vi "PMT_plus_Kiethley2450_and_2410.vi"() -> ()   [LabVIEW 2022 SP3]
uses:
  <vilib>/Utility/file.llb/Write Delimited Spreadsheet (string).vi
  <vilib>/Analysis/1siggen.llb/Ramp Pattern by Delta.vi
  <vilib>/Utility/file.llb/Write Delimited Spreadsheet (DBL).vi
  <vilib>/Analysis/NI_AALBase.lvlib
  C:/Users/Public/OneDrive/Desktop/test_save_lv22/Close.vi/Close Folder/Users/Public/OneDrive/Desktop/Keithley_2450_2470_1_4_0_LV2015_NewReadme2_2450-LV2015-1.4.0/Keithley 2450/Keithley 2450.lvlib
  D:/Download/Keithley 24XX/Keithley 24XX Folder/D/Download/Keithley 24XX/Keithley 24XX.lvlib
panel:
  out "current E field":dbl
  in  "d_t":dbl=-1.0 format="%#_13g"
  in  "d_b":dbl=-1.0 format="%#_13g"
  in  "E step (V/nm)":dbl=0.5 format="%#_13g"
  in  "E end (V/nm)":dbl=-1.0 format="%#_13g"
  in  "E start (V/nm)":dbl format="%#_13g"
  in  "Loop?":bool
  out "error out":errorcluster
  in  "use 2410":bool
  in  "use 2450?":bool=TRUE
  out "Set voltage 2410":dbl=-0.0
  out "current 2450":dbl=2.5622937e-12 format="%e"
  out "actual voltage 2410":dbl format="%0.2f"
  out "current 2410":dbl format="%e"
  in  "Compliance  Level 2410 (0.1)":dbl=1e-08
  in  "VISA resource name 2410":refnum<visa-resource-name>
  out "Serial Configuration":T1={"Baud Rate"=9600, "Parity"=0, "Data Bits"=8, "Stop Bits"=10, "Flow Control"=0} {"Flow Control" items=["None", "XON/XOFF", "RTS/CTS", "XON/XOFF & RTS/CTS", "DTR/DSR", "XON/XOFF & DTR/DSR"]; "Stop Bits" items=["1.0"=10, "1.5"=15, "2.0"=20]; "Data Bits" items=["7"=7, "8"=8]; "Parity" items=["None", "Odd", "Even", "Mark", "Space"]; "Baud Rate" items=["300"=300, "600"=600, "1200"=1200, "2400"=2400, "4800"=4800, "9600"=9600, "19200"=19200]}
  in  "Use PMT?":bool=TRUE
  out "XY Graph":cluster{dbl[], dbl[]}(graph)={[-1.0, -0.5, 0.0], [45.5, 47.5, 49.0]}
  out "Actual Voltage 2450":dbl
  in  "Num Current Meas":i32=20
  in  "Path":path=path "C:/Users/Public/OneDrive/Desktop/test.txt"
  in  "error in (no error)":errorcluster
  in  "VISA resource name":refnum<visa-resource-name>="GPIB0::1::INSTR"
  out "Set Voltage 2450":dbl
  in  "Step Size (V)":dbl=0.5 format="%#_13g"
  in  "End V":dbl=-1.0 format="%#_13g"
  in  "Start V":dbl format="%#_13g"
  in  "Source Limit Level (0.1)":dbl=1e-08
  out "standard deviation":dbl
  out "mean":dbl=49.0
  out "data":u32[](array[numeric])=[49, 49]
  out "OLD":bool
  out "DB":u32[](array[numeric])=[49, 0, 0, 0, 0, 0, 0, 0, 0, 0, 0, 0, 0, 0, 0, 0]
  out "Overload":i32
  out "Gate Number":i32=1
  in  "Correction":bool=TRUE
  out "Num Gates Read":i32=2
  out "Gate Time Read":i32=100 caption="Gate time Read"
  out "Num Gates Set":i32=2
  out "Gate Time Set":i32=100
  out "PowerD":i32 caption="Power\nRead Data"
  out "Handle Number":i32=173123648
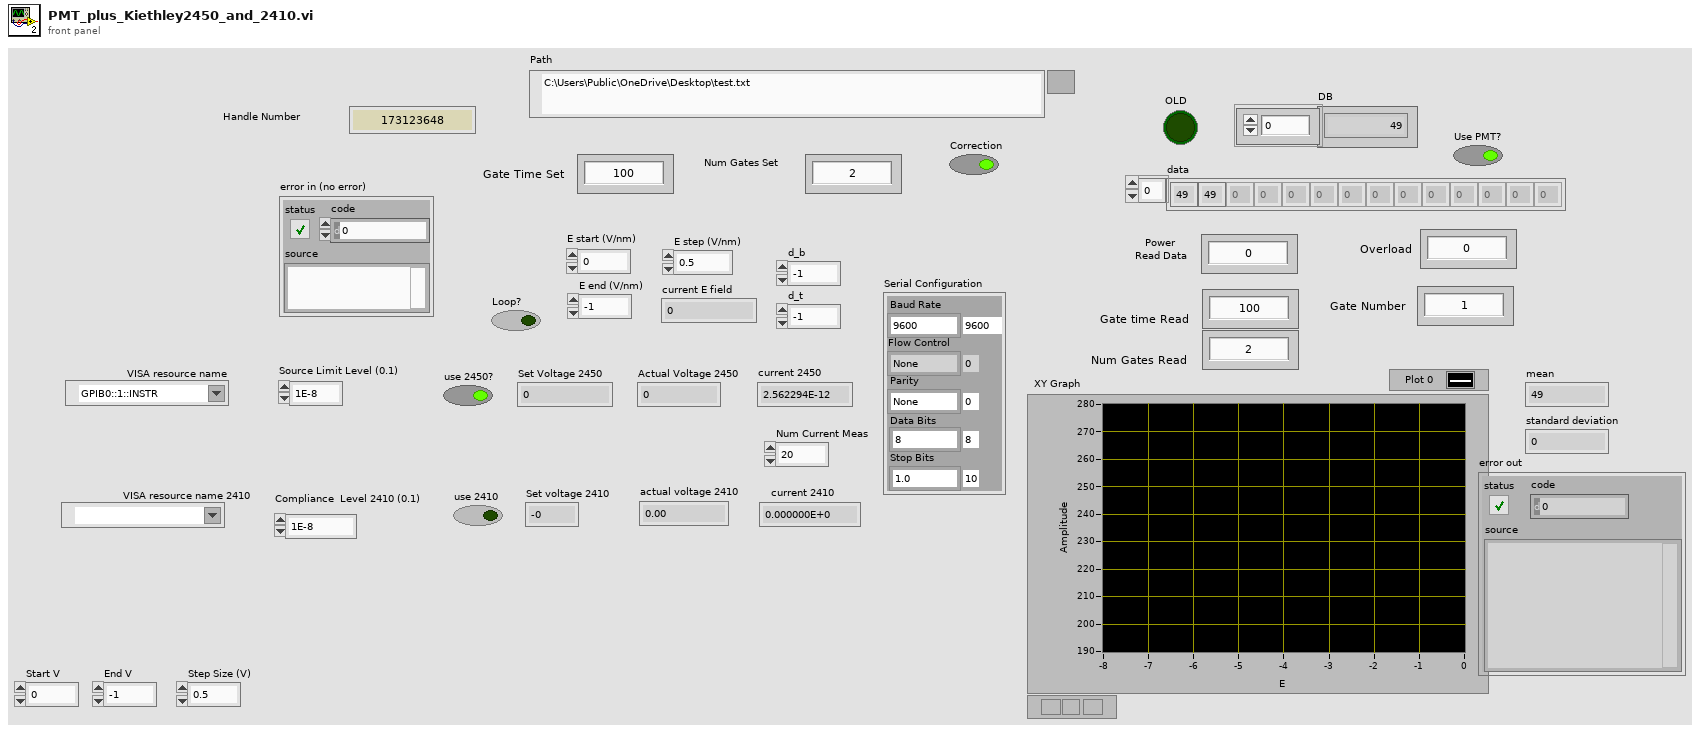
[diagram p1: front panel]
types:
  T1 = cluster{"Baud Rate":u32, "Parity":u16, "Data Bits":u16, "Stop Bits":u16, "Flow Control":u16}
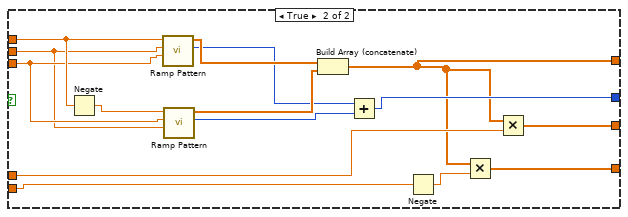
[diagram p2: hidden frame]
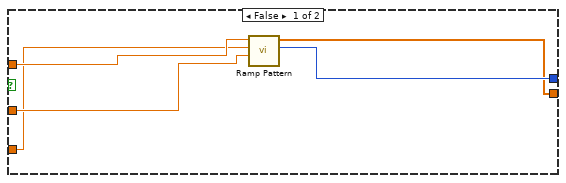
[diagram p3: hidden frame]
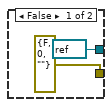
[diagram p4: hidden frame]
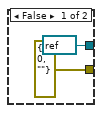
[diagram p5: hidden frame]
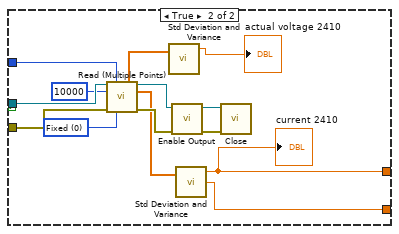
[diagram p6: hidden frame]
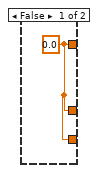
[diagram p7: hidden frame]
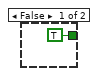
[diagram p8: hidden frame]
diagram:
  n1 = flat-sequence {
    tunnel: [w27] -> w8
    tunnel: [w15] -> w7
    tunnel: ["Path"] -> w5
    tunnel: ["use 2410"] -> w4
    tunnel: [w11] -> w3
    tunnel: [w10] -> w2
    tunnel: [w9] -> w1
    tunnel: w8 -> [w93]
    tunnel: w7 -> [w92]
    tunnel: [w91] -> w6
    tunnel: w5 -> [w90]
    tunnel: w4 -> [w85]
    tunnel: w3 -> [w84]
    tunnel: w2 -> [w83]
    tunnel: w1 -> [w82]
    tunnel: w6 -> [w575]
    frame #0 {
      # "open PMT and turn on power"
      n2 = call "Open.vi"("Serial Number"="30430219") -> ("Handle Number"=w31:i32)  [unwired: 9 in, 1 out]
      "Handle Number" <- w31
      n3 = case shown="False" "Loop?" {
        tunnel: "E step (V/nm)" -> [w46 w61]
        tunnel: "E end (V/nm)" -> [w45 w58]
        tunnel: "E start (V/nm)" -> [w44 w59]
        tunnel: [w43 w55] -> w15
        tunnel: "d_t" -> [w38 w49]
        tunnel: "d_b" -> [w42 w52]
        tunnel: [w41 w51] -> w11
        tunnel: [w40 w50] -> w10
        tunnel: [w37 w47] -> w9
        frame False {
          n4 = call-poly <vilib>:"Ramp Pattern.vi"("start"=w44, "end"=w45, "delta"=w46) -> ("samples"=w43:i32, "Ramp Pattern"=w37:dbl[])  [unwired: 6 in, 1 out]
          n5 = Negate(x=w38) -> (-x=w39:dbl)
          n6 = Multiply(x=w37, y=w39) -> (x*y=w40:dbl[])
          n7 = Multiply(x=w37, y=w42) -> (x*y=w41:dbl[])
        }
        frame True {
          n8 = Negate(x=w61) -> (-x=w60:dbl)
          n9 = call-poly <vilib>:"Ramp Pattern.vi"("start"=w59, "end"=w58, "delta"=w61) -> ("samples"=w54:i32, "Ramp Pattern"=w57:dbl[])  [unwired: 6 in, 1 out]
          n10 = call-poly <vilib>:"Ramp Pattern.vi"("start"=w58, "end"=w59, "delta"=w60) -> ("samples"=w53:i32, "Ramp Pattern"=w56:dbl[])  [unwired: 6 in, 1 out]
          n11 = Build Array (concatenate)(w57, w56) -> (w47:dbl[])
          n12 = Add(x=w54, y=w53) -> (x+y=w55:i32)
          n13 = Negate(x=w49) -> (-x=w48:dbl)
          n14 = Multiply(x=w47, y=w48) -> (x*y=w50:dbl[])
          n15 = Multiply(x=w47, y=w52) -> (x*y=w51:dbl[])
        }
      }
      n16 = Boolean To (0,1)(Boolean="Use PMT?") -> (0, 1=w32:i16)
      n17 = call "Read HV.vi"("handle"=w31) -> ("HV out"=w30:i32, "handle out"=w34:i32)  [unwired: 8 in, 1 out]
      n18 = case shown="True" "Loop?" {
        tunnel: "Start V" -> [w63 w74]
        tunnel: "End V" -> [w62 w72]
        tunnel: [w65 w71] -> _
        tunnel: [w66 w70] -> _
        tunnel: "Step Size (V)" -> [w64 w68]
        frame False {
          n19 = call-poly <vilib>:"Ramp Pattern.vi"("start"=w63, "end"=w62, "delta"=w64) -> ("samples"=w66:i32, "Ramp Pattern"=w65:dbl[])  [unwired: 6 in, 1 out]
        }
        frame True {
          w69 = -1.0
          n20 = Multiply(x=w68, y=w69) -> (x*y=w67:dbl)
          n21 = Multiply(x=w72, y=w69) -> (x*y=w73:dbl)
          n22 = call-poly <vilib>:"Ramp Pattern.vi"("start"=w74, "end"=w72, "delta"=w68) -> ("samples"=w78:i32, "Ramp Pattern"=w75:dbl[])  [unwired: 6 in, 1 out]
          n23 = call-poly <vilib>:"Ramp Pattern.vi"("start"=w73, "end"=w74, "delta"=w68) -> ("samples"=w81:i32, "Ramp Pattern"=w77:dbl[])  [unwired: 6 in, 1 out]
          n24 = call-poly <vilib>:"Ramp Pattern.vi"("start"=w72, "end"=w73, "delta"=w67) -> ("samples"=w79:i32, "Ramp Pattern"=w76:dbl[])  [unwired: 6 in, 1 out]
          n25 = Add(x=w78, y=w79) -> (x+y=w80:i32)
          n26 = Build Array (concatenate)(w75, w76, w77) -> (w71:dbl[])
          n27 = Add(x=w80, y=w81) -> (x+y=w70:i32)
        }
      }
      n28 = local write "PowerD"(w30) -> ()
      n29 = To Long Integer(number=w32) -> (32bit integer=w33:i32)
      n30 = call "Set HV.vi"("HV"=w33, "handle"=w34) -> ("handle out"=w36:i32)  [unwired: 8 in, 1 out]
      n31 = call "Read HV.vi"("handle"=w36) -> ("HV out"=w35:i32, "handle out"=w27:i32)  [unwired: 8 in, 1 out]
      n32 = Build Array("# SetVoltage2450(V) ActualVoltage2450(V) CountsMean CountsStd Current2450(uA) Current2450Std(uA) Current2410(uA) Current2410Std(uA)") -> (w22:string[])
      n33 = local write "PowerD"(w35) -> ()
      n34 = call-poly <vilib>:"Write Delimited Spreadsheet.vi"("file path (dialog if empty)"="Path", "1D data"=w22, "append to file? (new file:F)"=TRUE) -> ()  [unwired: 11 in, 2 out]
    }
    frame #1 {
      w88 = 0
      w89 = 0
      n35 = Initialize Array(w88, w88) -> (w87:i32[])
      n36 = Initialize Array(w89, w89) -> (w86:i32[])
      n37 = for {
        N: w92 -> [_]
        tunnel: w84 -> [w136] mode=indexing
        tunnel: w93 -> [w135]
        tunnel: [w134] -> w91
        tunnel: w90 -> [w133]
        shift-right: [w120] -> _
        shift-left: w86 -> [w128]
        shift-right: [w121] -> _
        shift-left: w87 -> [w127]
        tunnel: w85 -> [w98]
        tunnel: w83 -> [w95] mode=indexing
        tunnel: w82 -> [w94] mode=indexing
        n38 = flat-sequence {
          tunnel: w127 -> [w153]
          tunnel: w128 -> [w154]
          tunnel: w136 -> [w142]
          tunnel: [w142] -> w119
          tunnel: [w154] -> w117
          tunnel: [w153] -> w115
          tunnel: [w149] -> w113
          tunnel: [w148] -> w111
          tunnel: [w145] -> w107
          tunnel: [w144] -> w105
          tunnel: ["Num Current Meas"] -> w103
          tunnel: ["use 2450?"] -> w99
          tunnel: w98 -> [w138]
          tunnel: [w138] -> w96
          tunnel: w95 -> [w137]
          tunnel: w119 -> [w217]
          tunnel: [w217] -> w118
          tunnel: w117 -> [w216]
          tunnel: [w216] -> w116
          tunnel: w115 -> [w215]
          tunnel: [w215] -> w114
          tunnel: w113 -> [w214]
          tunnel: [w214] -> w112
          tunnel: w111 -> [w213]
          tunnel: [w213] -> w110
          tunnel: [w212] -> w108
          tunnel: w107 -> [w212]
          tunnel: [w211] -> w106
          tunnel: w105 -> [w211]
          tunnel: [w210] -> w104
          tunnel: w103 -> [w210]
          tunnel: [w209] -> w100
          tunnel: w99 -> [w209]
          tunnel: [w208] -> w97
          tunnel: w96 -> [w208]
          tunnel: [w231] -> w132
          tunnel: [w232] -> w131
          tunnel: [w222] -> w130
          tunnel: [w231] -> w129
          tunnel: [w230] -> w126
          tunnel: [w229] -> w125
          tunnel: w118 -> [w231]
          tunnel: w116 -> [w230]
          tunnel: w114 -> [w229]
          tunnel: w112 -> [w225]
          tunnel: w110 -> [w226]
          tunnel: [w223] -> w109
          tunnel: w108 -> [w228]
          tunnel: w106 -> [w227]
          tunnel: w104 -> [w224]
          tunnel: [w221] -> w102
          tunnel: [w220] -> w101
          tunnel: w100 -> [w219]
          tunnel: w97 -> [w218]
          tunnel: w135 -> [w289]
          tunnel: w133 -> [w287]
          tunnel: w132 -> [w286]
          tunnel: w131 -> [w285]
          tunnel: w130 -> [w284]
          tunnel: w129 -> [w282]
          tunnel: w126 -> [w281]
          tunnel: w125 -> [w280]
          tunnel: [w288] -> w124
          tunnel: [w279] -> w123
          tunnel: [w278] -> w122
          tunnel: w109 -> [w277]
          tunnel: w102 -> [w275]
          tunnel: w101 -> [w274]
          tunnel: [w572] -> w120
          tunnel: [w573] -> w121
          tunnel: [w574] -> w134
          tunnel: w124 -> [w574]
          tunnel: w123 -> [w573]
          tunnel: w122 -> [w572]
          frame #0 {
            w140 = TRUE
            w146 = FALSE
            n39 = case shown="True" "use 2450?" {
              tunnel: "VISA resource name" -> [_ w198]
              tunnel: "error in (no error)" -> [_ w197]
              tunnel: TRUE -> [_ w193]
              tunnel: [errorcluster {"status"=FALSE, "code"=0, "source"=""} ("error out") w192] -> w149
              tunnel: [refnum<visa-resource-name> refnum ("VISA resource name out") w191] -> w148
              tunnel: w146 -> [_ w190]
              tunnel: "Num Current Meas" -> [_ w181]
              tunnel: w142 -> [_ w180]
              tunnel: "Source Limit Level (0.1)" -> [_ w179]
              tunnel: w140 -> [_ w178]
              tunnel: w140 -> [_ w177]
              frame False {
              }
              frame True {
                w194 = 1
                w196 = 0
                n40 = call "Initialize.vi"("error in (no error)"=w197, "Reset (True)"=w190, "ID Query (True)"=w193, "VISA resource name"=w198) -> ("error out"=w188:errorcluster, "VISA resource name out"=w189:refnum<visa-resource-name>)  [unwired: 6 in]
                n41 = call "Clear Buffer.vi"("VISA resource name"=w189, "error in (no error)"=w188) -> ("VISA resource name out"=w186:refnum<visa-resource-name>, "error out"=w187:errorcluster)  [unwired: 12 in]
                n42 = call "Configure Measurement Range.vi"("error in (no error)"=w187, "Enable Auto Range (T:Enable)"=w177, "Function (0: Volts)"=w196, "VISA resource name"=w186) -> ("error out"=w206:errorcluster, "VISA resource name out"=w205:refnum<visa-resource-name>)  [unwired: 6 in]
                n43 = call "Configure Measurement Range.vi"("error in (no error)"=w206, "Enable Auto Range (T:Enable)"=w178, "Function (0: Volts)"=w194, "VISA resource name"=w205) -> ("error out"=w202:errorcluster, "VISA resource name out"=w199:refnum<visa-resource-name>)  [unwired: 6 in]
                n44 = call "Configure Output.vi"("VISA resource name"=w199, "Source Level (0)"=w180, "Source Limit Level (0.1)"=w179, "error in (no error)"=w202) -> ("VISA resource name out"=w200:refnum<visa-resource-name>, "error out"=w203:errorcluster)  [unwired: 10 in]
                n45 = call "Configure Source Function.vi"("error in (no error)"=w203, "Function (0: Volts)"=w196, "VISA resource name"=w200) -> ("error out"=w204:errorcluster, "VISA resource name out"=w201:refnum<visa-resource-name>)  [unwired: 7 in]
                n46 = call "Configure Measurement Function.vi"("error in (no error)"=w204, "Function (0: Volts)"=w194, "VISA resource name"=w201) -> ("error out"=w182:errorcluster, "VISA resource name out"=w185:refnum<visa-resource-name>)  [unwired: 7 in]
                n47 = call "Set Measurement Count.vi"("error in (no error)"=w182, "Measurement Count (1)"=w181, "VISA resource name"=w185) -> ("error out"=w183:errorcluster, "VISA resource name out"=w184:refnum<visa-resource-name>)  [unwired: 7 in]
                n48 = call "Enable Output.vi"("error in (no error)"=w183, "Enable Output (T: Enable)"=TRUE, "VISA resource name"=w184) -> ("error out"=w192:errorcluster, "VISA resource name out"=w191:refnum<visa-resource-name>)  [unwired: 7 in]
              }
            }
            n49 = case shown="True" w138 {
              tunnel: "VISA resource name 2410" -> [_ w174]
              tunnel: w146 -> [_ w173]
              tunnel: [refnum<visa-resource-name> refnum ("VISA resource name out") w160] -> w145
              tunnel: [errorcluster {"status"=FALSE, "code"=0, "source"=""} ("error out") w159] -> w144
              tunnel: w137 -> [_ w158]
              tunnel: w140 -> [_ w157]
              frame False {
              }
              frame True {
                w162 = u16 0 items=["Voltage", "Current"] ("Source Mode  (0: Voltage)")
                w163 = u16 1 items=["Volts", "Current", "Resistance"] ("Function (0: Volts)")
                w164 = u16 0 items=["Volts", "Current", "Resistance"] ("Function (0: Volts)")
                n50 = call "Initialize.vi"("Reset (True)"=w173, "VISA resource name"=w174) -> ("error out"=w171:errorcluster, "VISA resource name out"=w172:refnum<visa-resource-name>)  [unwired: 8 in]
                n51 = call "Configure Measurement.vi"("error in (no error)"=w171, "Enable Auto Range (T:Enable)"=w157, "Function (0: Volts)"=w164, "VISA resource name"=w172) -> ("error out"=w170:errorcluster, "VISA resource name out"=w169:refnum<visa-resource-name>)  [unwired: 6 in]
                n52 = call "Configure Measurement.vi"("error in (no error)"=w170, "Enable Auto Range (T:Enable)"=w157, "Function (0: Volts)"=w163, "VISA resource name"=w169) -> ("error out"=w167:errorcluster, "VISA resource name out"=w168:refnum<visa-resource-name>)  [unwired: 6 in]
                n53 = call "Configure Output.vi"("Source Mode  (0: Voltage)"=w162, "error in (no error)"=w167, "Compliance  Level (0.1)"="Compliance  Level 2410 (0.1)", "Output Level (0)"=w158, "VISA resource name"=w168) -> ("error out"=w165:errorcluster, "VISA resource name out"=w166:refnum<visa-resource-name>)  [unwired: 5 in]
                n54 = call "Enable Output.vi"("error in (no error)"=w165, "VISA resource name"=w166) -> ("error out"=w159:errorcluster, "VISA resource name out"=w160:refnum<visa-resource-name>)  [unwired: 8 in]
              }
            }
            "Set Voltage 2450" <- w142
            "Set voltage 2410" <- w137
          }
          frame #1 {
            n55 = Wait (ms)(milliseconds to wait=u32 100) -> ()  [unwired: 1 out]
          }
          frame #2 {
            n56 = case shown="False" w218 {
              tunnel: w228 -> [_ w247]
              tunnel: w227 -> [_ w246]
              tunnel: w224 -> [_ w237]
              tunnel: [w233 w235] -> w221
              tunnel: [w233 w234] -> w220
              frame False {
                w233 = 0.0 ("mean")
              }
              frame True {
                w245 = u16 0 items=["Fixed", "Sweep", "List"] ("Output Mode (0: Fixed)")
                n57 = call "Read (Multiple Points).vi"("VISA resource name"=w247, "Sample Count (1)"=w237, "Timeout (10000 ms)"=10000, "error in (no error)"=w246, "Output Mode (0: Fixed)"=w245) -> ("Voltage"=w238:sgl[], "VISA resource name out"=w243:refnum<visa-resource-name>, "Current"=w239:sgl[], "error out"=w240:errorcluster)  [unwired: 4 in, 3 out]
                n58 = call <vilib>:"Std Deviation and Variance.vi"("X"=w238) -> ("mean"=→"actual voltage 2410":dbl)  [unwired: 1 in, 2 out]
                n59 = call "Enable Output.vi"("error in (no error)"=w240, "VISA resource name"=w243) -> ("error out"=w241:errorcluster, "VISA resource name out"=w242:refnum<visa-resource-name>)  [unwired: 8 in]
                n60 = call <vilib>:"Std Deviation and Variance.vi"("X"=w239) -> ("mean"=w235:dbl, "standard deviation"=w234:dbl)  [unwired: 1 in, 1 out]
                "current 2410" <- w235
                n61 = call "Close.vi"("error in (no error)"=w241, "VISA resource name"=w242) -> ()  [unwired: 9 in, 1 out]
              }
            }
            n62 = case shown="True" w219 {
              tunnel: [w248 w270] -> w232
              tunnel: w226 -> [_ w269]
              tunnel: w225 -> [_ w268]
              tunnel: w224 -> [_ w265]
              tunnel: [w248 w255] -> w223
              tunnel: [w248 w253] -> w222
              frame False {
                w248 = 0.0 ("Voltage Level Out")
              }
              frame True {
                w252 = 1000000
                n63 = call "Make Reading and Store in Buffer.vi"("VISA resource name"=w269, "error in (no error)"=w268) -> ("VISA resource name out"=w267:refnum<visa-resource-name>, "error out"=w266:errorcluster)  [unwired: 12 in]
                n64 = call "Read (Multiple Points).vi"("VISA resource name"=w267, "Start Index (1)"=u32 1, "End Index (1)"=w265, "error in (no error)"=w266) -> ("VISA resource name out"=w258:refnum<visa-resource-name>, "Data out"=w263:string, "error out"=w257:errorcluster)  [unwired: 9 in]
                n65 = call "Get Source Level.vi"("error in (no error)"=w257, "VISA resource name"=w258) -> ("error out"=w272:errorcluster, "Voltage Level Out"=w270:dbl, "VISA resource name out"=w273:refnum<visa-resource-name>)  [unwired: 6 in, 1 out]
                "Actual Voltage 2450" <- w270
                n66 = Spreadsheet String To Array(delimiter (Tab)=",", format string="%s", spreadsheet string=w263, array type (2D Dbl)=dbl[] []) -> (array=w259:dbl[])
                n67 = call "Enable Output.vi"("error in (no error)"=w272, "Enable Output (T: Enable)"=TRUE, "VISA resource name"=w273) -> ("error out"=w249:errorcluster, "VISA resource name out"=w250:refnum<visa-resource-name>)  [unwired: 7 in]
                n68 = call "Close.vi"("error in (no error)"=w249, "VISA resource name"=w250) -> ("error out"=→"error out":errorcluster)  [unwired: 9 in]
                n69 = call <vilib>:"Std Deviation and Variance.vi"("X"=w259) -> ("mean"=w254:dbl, "standard deviation"=w256:dbl)  [unwired: 1 in, 1 out]
                "current 2450" <- w254
                n70 = Multiply(x=w254, y=w252) -> (x*y=w253:dbl)
                n71 = Multiply(x=w256, y=w252) -> (x*y=w255:dbl)
              }
            }
          }
          frame #3 {
            n72 = case shown="True" FALSE {
              tunnel: [TRUE w293] -> w283
              tunnel: w282 -> [_ w292]
              frame False {
              }
              frame True {
                n73 = Quotient & Remainder(x=w292, y=2) -> (x-y*floor(x/y)=w294:dbl)  [unwired: 1 out]
                n74 = Equal To 0?(x=w294) -> (x = 0?=w293:bool)
              }
            }
            n75 = case shown="True" w283 {
              tunnel: w289 -> [w297 w343]
              tunnel: [w297 w342] -> w288
              tunnel: w287 -> [_ w341]
              tunnel: w286 -> [_ w340]
              tunnel: w285 -> [_ w339]
              tunnel: w284 -> [_ w338]
              tunnel: w281 -> [w296 w337]
              tunnel: w280 -> [w295 w325]
              tunnel: [w296 w313] -> w279
              tunnel: [w295 w312] -> w278
              tunnel: w277 -> [_ w311]
              tunnel: w275 -> [_ w299]
              tunnel: w274 -> [_ w298]
              frame False {
              }
              frame True {
                n76 = flat-sequence {
                  tunnel: [w402] -> w396
                  tunnel: [w400] -> w395
                  tunnel: [w401] -> w394
                  tunnel: w340 -> [w402]
                  tunnel: w339 -> [w401]
                  tunnel: w338 -> [w400]
                  tunnel: w337 -> [w399]
                  tunnel: [w399] -> w326
                  tunnel: w325 -> [w398]
                  tunnel: [w398] -> w318
                  tunnel: w311 -> [w397]
                  tunnel: [w397] -> w307
                  tunnel: [w409] -> w393
                  tunnel: w343 -> [w409]
                  tunnel: [w408] -> w392
                  tunnel: w396 -> [w408]
                  tunnel: [w407] -> w391
                  tunnel: w395 -> [w407]
                  tunnel: [w406] -> w390
                  tunnel: w394 -> [w406]
                  tunnel: [w405] -> w327
                  tunnel: w326 -> [w405]
                  tunnel: [w404] -> w319
                  tunnel: w318 -> [w404]
                  tunnel: [w403] -> w308
                  tunnel: w307 -> [w403]
                  tunnel: w393 -> [w423]
                  tunnel: [w418] -> w389
                  tunnel: [w416] -> w388
                  tunnel: w392 -> [w416]
                  tunnel: [w415] -> w387
                  tunnel: w391 -> [w415]
                  tunnel: [w414] -> w386
                  tunnel: w390 -> [w414]
                  tunnel: [w413] -> w328
                  tunnel: w327 -> [w413]
                  tunnel: [w412] -> w320
                  tunnel: w319 -> [w412]
                  tunnel: [w411] -> w309
                  tunnel: w308 -> [w411]
                  tunnel: [w432] -> w385
                  tunnel: w389 -> [w434]
                  tunnel: [w429] -> w384
                  tunnel: w388 -> [w429]
                  tunnel: w387 -> [w428]
                  tunnel: [w428] -> w383
                  tunnel: [w427] -> w382
                  tunnel: w386 -> [w427]
                  tunnel: [w426] -> w329
                  tunnel: w328 -> [w426]
                  tunnel: [w425] -> w321
                  tunnel: w320 -> [w425]
                  tunnel: [w424] -> w310
                  tunnel: w309 -> [w424]
                  tunnel: w385 -> [w447]
                  tunnel: [w447] -> w381
                  tunnel: [w443] -> w380
                  tunnel: [w443] -> w379
                  tunnel: [w442] -> w378
                  tunnel: w384 -> [w442]
                  tunnel: [w441] -> w377
                  tunnel: w383 -> [w441]
                  tunnel: w382 -> [w440]
                  tunnel: [w440] -> w376
                  tunnel: [w439] -> w330
                  tunnel: w329 -> [w439]
                  tunnel: [w438] -> w322
                  tunnel: w321 -> [w438]
                  tunnel: w310 -> [w437]
                  tunnel: [w437] -> w303
                  tunnel: w381 -> [w460]
                  tunnel: [w456] -> w375
                  tunnel: w380 -> [w455]
                  tunnel: w379 -> [w454]
                  tunnel: [w455] -> w374
                  tunnel: [w454] -> w373
                  tunnel: w378 -> [w453]
                  tunnel: [w453] -> w372
                  tunnel: [w452] -> w371
                  tunnel: w377 -> [w452]
                  tunnel: [w451] -> w370
                  tunnel: w376 -> [w451]
                  tunnel: [w450] -> w331
                  tunnel: w330 -> [w450]
                  tunnel: [w449] -> w323
                  tunnel: w322 -> [w449]
                  tunnel: [w448] -> w304
                  tunnel: w303 -> [w448]
                  tunnel: [w473] -> w369
                  tunnel: w375 -> [w472]
                  tunnel: w374 -> [w471]
                  tunnel: w373 -> [w470]
                  tunnel: [w469] -> w368
                  tunnel: [w466] -> w367
                  tunnel: w372 -> [w466]
                  tunnel: [w465] -> w366
                  tunnel: w371 -> [w465]
                  tunnel: w370 -> [w464]
                  tunnel: [w464] -> w365
                  tunnel: [w463] -> w332
                  tunnel: w331 -> [w463]
                  tunnel: [w462] -> w324
                  tunnel: w323 -> [w462]
                  tunnel: [w461] -> w305
                  tunnel: w304 -> [w461]
                  tunnel: w369 -> [w527]
                  tunnel: [w526] -> w364
                  tunnel: [w525] -> w363
                  tunnel: w368 -> [w525]
                  tunnel: w367 -> [w524]
                  tunnel: [w524] -> w362
                  tunnel: [w523] -> w361
                  tunnel: w366 -> [w523]
                  tunnel: [w522] -> w360
                  tunnel: w365 -> [w522]
                  tunnel: [w521] -> w333
                  tunnel: w332 -> [w521]
                  tunnel: w324 -> [w520]
                  tunnel: [w520] -> w315
                  tunnel: [w519] -> w306
                  tunnel: w305 -> [w519]
                  tunnel: w364 -> [w534]
                  tunnel: w363 -> [w535]
                  tunnel: [w535] -> w359
                  tunnel: [w534] -> w358
                  tunnel: [w533] -> w357
                  tunnel: w362 -> [w533]
                  tunnel: w361 -> [w532]
                  tunnel: [w532] -> w356
                  tunnel: w360 -> [w531]
                  tunnel: [w531] -> w355
                  tunnel: [w530] -> w334
                  tunnel: w333 -> [w530]
                  tunnel: [w529] -> w316
                  tunnel: w315 -> [w529]
                  tunnel: w306 -> [w528]
                  tunnel: [w528] -> w300
                  tunnel: [w543] -> w354
                  tunnel: w359 -> [w543]
                  tunnel: [w542] -> w353
                  tunnel: w358 -> [w542]
                  tunnel: [w541] -> w352
                  tunnel: w357 -> [w541]
                  tunnel: [w540] -> w351
                  tunnel: w356 -> [w540]
                  tunnel: [w539] -> w350
                  tunnel: w355 -> [w539]
                  tunnel: [w538] -> w335
                  tunnel: w334 -> [w538]
                  tunnel: [w537] -> w317
                  tunnel: w316 -> [w537]
                  tunnel: [w536] -> w301
                  tunnel: w300 -> [w536]
                  tunnel: w354 -> [w553]
                  tunnel: [w552] -> w349
                  tunnel: [w551] -> w348
                  tunnel: [w550] -> w347
                  tunnel: w353 -> [w550]
                  tunnel: [w549] -> w346
                  tunnel: w352 -> [w549]
                  tunnel: [w548] -> w345
                  tunnel: w351 -> [w548]
                  tunnel: [w547] -> w344
                  tunnel: w350 -> [w547]
                  tunnel: [w546] -> w336
                  tunnel: w335 -> [w546]
                  tunnel: w317 -> [w545]
                  tunnel: [w545] -> w314
                  tunnel: [w544] -> w302
                  tunnel: w301 -> [w544]
                  tunnel: w349 -> [w560]
                  tunnel: w348 -> [w568]
                  tunnel: [w570] -> w342
                  tunnel: w347 -> [w570]
                  tunnel: w341 -> [w569]
                  tunnel: w346 -> [w563]
                  tunnel: w345 -> [w566]
                  tunnel: w344 -> [w559]
                  tunnel: w336 -> [w562]
                  tunnel: w314 -> [w561]
                  tunnel: [w558] -> w313
                  tunnel: [w557] -> w312
                  tunnel: w302 -> [w556]
                  tunnel: w299 -> [w555]
                  tunnel: w298 -> [w554]
                  frame #0 {
                  }
                  frame #1 {
                    n77 = Wait (ms)(milliseconds to wait=u32 200) -> ()  [unwired: 1 out]
                  }
                  frame #2 {
                    # "set gate time"
                    n78 = local read "Gate Time Set"() -> (w420:i32)
                    n79 = Wait (ms)(milliseconds to wait=u32 200) -> ()  [unwired: 1 out]
                    n80 = To Long Integer(number=w420) -> (32bit integer=w421:i32)
                    n81 = call "Set IT.vi"("IT"=w421, "handle"=w423) -> ("handle out"=w422:i32)  [unwired: 8 in, 1 out]
                    n82 = call "Read IT.vi"("handle"=w422) -> ("IT out"=w419:i32, "handle out"=w418:i32)  [unwired: 8 in, 1 out]
                    n83 = local write "Gate Time Read"(w419) -> ()
                  }
                  frame #3 {
                    # "set number of gates"
                    n84 = local read "Num Gates Set"() -> (w436:i32)
                    n85 = Wait (ms)(milliseconds to wait=u32 200) -> ()  [unwired: 1 out]
                    n86 = To Long Integer(number=w436) -> (32bit integer=w435:i32)
                    n87 = call "Set RN.vi"("RN"=w435, "handle"=w434) -> ("handle out"=w433:i32)  [unwired: 8 in, 1 out]
                    n88 = call "Read RN.vi"("handle"=w433) -> ("RN out"=w431:i32, "handle out"=w432:i32)  [unwired: 8 in, 1 out]
                    n89 = local write "Num Gates Read"(w431) -> ()
                  }
                  frame #4 {
                    # "gate number data"
                    # "count data"
                    n90 = local write "Gate Number"(0) -> ()
                    n91 = Initialize Array(u32 0, 0 ("次元サイズ")) -> (w443:u32[])
                  }
                  frame #5 {
                    n92 = Boolean To (0,1)(Boolean="Correction") -> (0, 1=w459:i16)
                    n93 = To Long Integer(number=w459) -> (32bit integer=w458:i32)
                    n94 = call "Count Start.vi"("Correction"=w458, "handle"=w460) -> ("handle out"=w456:i32)  [unwired: 8 in, 1 out]
                  }
                  frame #6 {
                    n95 = local read "Num Gates Read"() -> (w468:i32)
                    n96 = for {
                      N: w468 -> [_]
                      shift-right: [w474] -> w469
                      shift-left: w471 -> [w482]
                      shift-right: [w478] -> _
                      shift-left: w470 -> [w481]
                      tunnel: w472 -> [w483]
                      tunnel: [w484] -> w473
                      tunnel: [w474] -> w467
                      n97 = flat-sequence {
                        tunnel: [w494] -> w488
                        tunnel: [w493] -> w479
                        tunnel: [w492] -> w476
                        tunnel: w483 -> [w494]
                        tunnel: w482 -> [w493]
                        tunnel: w481 -> [w492]
                        tunnel: [w505] -> w487
                        tunnel: w488 -> [w504]
                        tunnel: [w499] -> w486
                        tunnel: [w498] -> w485
                        tunnel: [w497] -> w480
                        tunnel: w479 -> [w497]
                        tunnel: [w496] -> w477
                        tunnel: w476 -> [w496]
                        tunnel: [w495] -> w475
                        tunnel: w487 -> [w518]
                        tunnel: w486 -> [w513]
                        tunnel: w485 -> [w512]
                        tunnel: w480 -> [w510]
                        tunnel: w477 -> [w509]
                        tunnel: w475 -> [w508]
                        tunnel: [w518] -> w484
                        tunnel: [w511] -> w474
                        tunnel: [w506] -> w478
                        frame #0 {
                          n98 = Initialize Array(u32 0, 16 ("次元サイズ")) -> (w489:u32[])
                          n99 = local write "DB"(w489) -> ()
                        }
                        frame #1 {
                          # "read data"
                          n100 = local read "Gate Number"() -> (w503:i32)
                          n101 = local read "Overload"() -> (w502:i32)
                          n102 = local read "DB"() -> (w500:u32[])
                          n103 = call "Read Data.vi"("OLD"=w502, "DataBuf"=w500, "GateNum"=w503, "handle"=w504) -> ("OLD out"=w501:i32, "DataBuf out"=w498:u32[], "GateNum out"=w495:i32, "handle out"=w505:i32, "function return"=w499:u32)  [unwired: 3 in]
                          n104 = local write "Gate Number"(w495) -> ()
                          n105 = local write "DB"(w498) -> ()
                          n106 = local write "Overload"(w501) -> ()
                        }
                        frame #2 {
                          # "Pickup Tans Data!"
                          n107 = To Long Integer(number=w513) -> (32bit integer=w514:i32)
                          n108 = Build Array(w508) -> (w507:i32[])
                          n109 = local read "Overload"() -> (w516:i32)
                          n110 = Build Array (concatenate)(w509, w507) -> (w506:u32[])
                          n111 = Array Subset(array=w512, length=w514) -> (w515:u32[])  [unwired: 1 in]
                          n112 = Not Equal To 0?(x=w516) -> (x != 0?=→"OLD":bool)
                          n113 = Build Array (concatenate)(w510, w515) -> (w511:u32[])
                        }
                      }
                    }
                    "data" <- w467
                  }
                  frame #7 {
                    # "data"
                    n114 = call "Count Stop.vi"("handle"=w527) -> ("handle out"=w526:i32)  [unwired: 9 in, 1 out]
                  }
                  frame #8 {
                  }
                  frame #9 {
                  }
                  frame #10 {
                    n115 = call <vilib>:"Std Deviation and Variance.vi"("X"=w553) -> ("mean"=w552:dbl, "standard deviation"=w551:dbl)  [unwired: 1 in, 1 out]
                  }
                  frame #11 {
                    n116 = Build Array (concatenate)(w561, w559) -> (w558:dbl[])
                    n117 = Build Array(w563, w559, w560, w568, w566, w556, w555, w554) -> (w567:dbl[])
                    n118 = Build Array (concatenate)(w562, w560) -> (w557:dbl[])
                    n119 = call-poly <vilib>:"Write Delimited Spreadsheet.vi"("file path (dialog if empty)"=w569, "format (%.3f)"="%.10f", "1D data"=w567, "append to file? (new file:F)"=TRUE) -> ()  [unwired: 10 in, 2 out]
                    "mean" <- w560
                    "standard deviation" <- w568
                  }
                }
              }
            }
          }
          frame #4 {
            n120 = Bundle(w573, w572) -> (→"XY Graph":cluster{dbl[], dbl[]})  [unwired: 1 in]
          }
        }
        "current E field" <- w94
      }
    }
    frame #2 {
      # "turn off PMT and close"
      n121 = Boolean To (0,1)(Boolean=FALSE) -> (0, 1=w580:i16)
      n122 = To Long Integer(number=w580) -> (32bit integer=w579:i32)
      n123 = call "Set HV.vi"("HV"=w579, "handle"=w575) -> ("handle out"=w577:i32)  [unwired: 8 in, 1 out]
      n124 = call "Read HV.vi"("handle"=w577) -> ("HV out"=w581:i32, "handle out"=w576:i32)  [unwired: 8 in, 1 out]
      n125 = call "Close.vi"("Handle"=w576) -> ()  [unwired: 9 in, 2 out]
      n126 = local write "PowerD"(w581) -> ()
    }
  }
